vi "WSVCAP SHL Host TL SPI Write Cycle - Multiple DUTs - Common Data.vi"(0 "Data Out (Cycle Commands)":string[](array[string]), 5 "Post Command Delay":dbl[](array[numeric]) format="%#.0p s", 11 "error in":errorcluster, 13 "DUT Mask (All)":bool[](array[boolean])=[TRUE, TRUE, TRUE, TRUE, TRUE, TRUE, TRUE, TRUE, TRUE, TRUE, TRUE, TRUE, TRUE, TRUE, TRUE, TRUE]) -> (15 "error out":errorcluster)   [LabVIEW 2012]
panel:
  out "Socket Mask":u16=1 format="%02x"
  out "SPI Data Out [U8]":u8[][](array[numeric]) format="%02x"
  # "DUT 01"
  # "DUT 02"
  # "DUT 03"
  # "DUT 04"
  # "DUT 05"
  # "DUT 06"
  # "DUT 07"
  # "DUT 08"
  # "DUT 09"
  # "DUT 10"
  # "DUT 11"
  # "DUT 12"
  # "DUT 13"
  # "DUT 14"
  # "DUT 15"
  # "DUT 16"
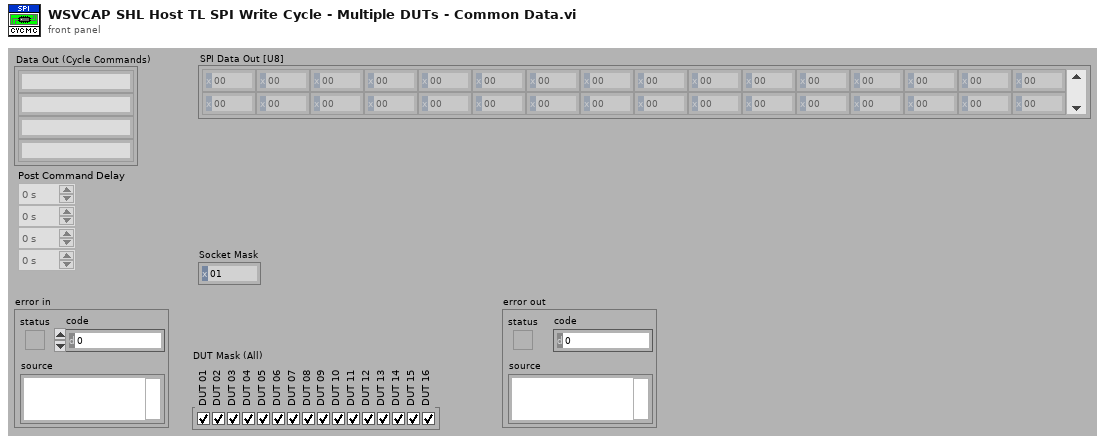
[diagram p1: front panel]
types:
  T1 = typedef "WSVCAP SHL Core System Cluster.ctl" = cluster{"Settings":T2, "FPGA Resource":tag, "Online":bool, "I2C Wait Ticks":u32, "SPI Wait Ticks":u32, "RFFE Wait Ticks":u32}
  T2 = typedef "WSVCAP SHL I2C Settings Cluster.ctl" = cluster{"FPGA Resource Name":string, "I2C Slave Address":u8, "I2C Clock Rate (Hz)":dbl, "SPI Clock Rate (Hz)":dbl, "RFFE Slave Address":u8, "RFFE Clock Rate (Hz)":dbl, "Simulate FPGA":bool}
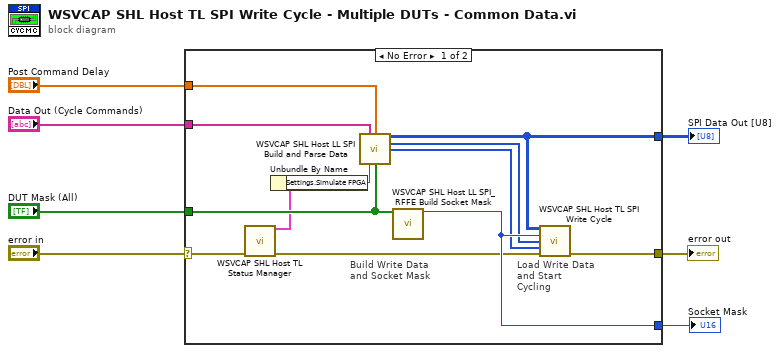
[diagram p0: block diagram]
diagram:
  n1 = case shown="No Error" "error in" {
    selector: "error in" -> [w12 _]
    tunnel: [w19 _] -> w7
    tunnel: [w17 _] -> w5
    tunnel: [w16 _] -> w4
    tunnel: "DUT Mask (All)" -> [w18 _]
    tunnel: "Post Command Delay" -> [w15 _]
    tunnel: "Data Out (Cycle Commands)" -> [w14 _]
    frame No Error {
      # "Load Write Data and Start Cycling"
      # "Build Write Data and Socket Mask"
      n2 = call "WSVCAP SHL Host TL Status Manager.vi"("error in"=w12) -> ("System Out"=w13:T1, "error out"=w11:errorcluster)  [unwired: 13 in]
      n3 = Unbundle By Name(w13) -> ("Settings.Simulate FPGA"=w10:bool)
      n4 = call "WSVCAP SHL Host LL SPI Build and Parse Data.vi"("Data Out (Cycle Commands)"=w14, "Post Command Delay"=w15, "Simulate FPGA (Cycle Only)"=w10, "DUT Mask (All)"=w18) -> ("SPI Data Out [U8]"=w17:u8[][], "CMD Lengths (Bits)"=w9:u8[], "CMD Delays (Ticks)"=w8:u32[])  [unwired: 8 in, 1 out]
      n5 = call "WSVCAP SHL Host LL SPI_RFFE Build Socket Mask.vi"("DUT Mask"=w18) -> ("Socket Mask [U16]"=w16:u16)  [unwired: 13 in, 1 out]
      n6 = call "WSVCAP SHL Host TL SPI Write Cycle.vi"("SPI Data Out"=w17, "Socket Mask"=w16, "Cycle CMD Lengths (bits)"=w9, "Cycle CMD Delay (ticks)"=w8, "error in"=w11) -> ("error out"=w19:errorcluster)  [unwired: 10 in]
    }
    frame Error {
    }
  }
  "error out" <- w7
  "SPI Data Out [U8]" <- w5
  "Socket Mask" <- w4
